vi "Set Bucket RequestPayment Configuration.vi"(4 "Region":T1, 7 "RequestPayment Configuration":T2, 8 "error in (no error)":errorcluster, 9 "Bucket":string) -> (0 "error out":errorcluster)   [LabVIEW 2015, in "LV Interface for Amazon S3.lvlib"]
doc: "This operation <B>sets the RequestPayment configuration</B> of a bucket. By default, <B>the bucket owner pays for downloads from the bucket</B>. This configuration parameter enables the bucket owner (only) to specify that the person requesting the download will be charged for the download."
uses:
  LV Interface for Amazon S3.lvlib
  Typedefs/AMZ_S3_API_RequestPaymentConfig.ctl
  Typedefs/AMZ_S3_Payer.ctl
  Typedefs/AMZ_S3_LocationConstraint.ctl
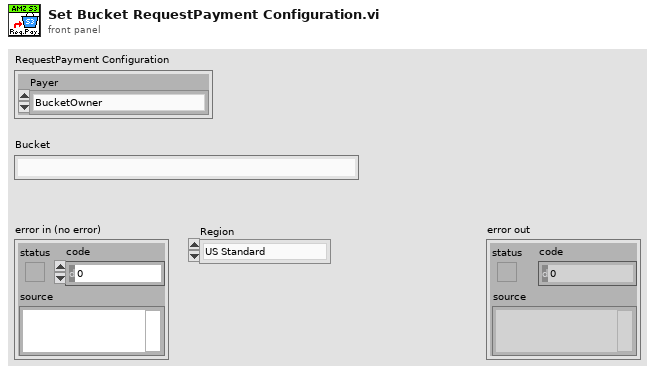
[diagram p1: front panel]
types:
  T1 = typedef "LV Interface for Amazon S3.lvlib/AMZ_S3_LocationConstraint.ctl" = enum16{"US Standard", "us-east-2", "us-west-1", "us-west-2", "ap-northeast-1", "ap-northeast-2", "ap-southeast-1", "ap-southeast-2", "ca-central-1", "eu-central-1", "eu-west-1", "eu-west-2", "sa-east-1"}
  T2 = typedef "LV Interface for Amazon S3.lvlib/AMZ_S3_API_RequestPaymentConfig.ctl" = cluster{"Payer":T3}
  T3 = typedef "LV Interface for Amazon S3.lvlib/AMZ_S3_Payer.ctl" = enum16{"BucketOwner", "Requester"}
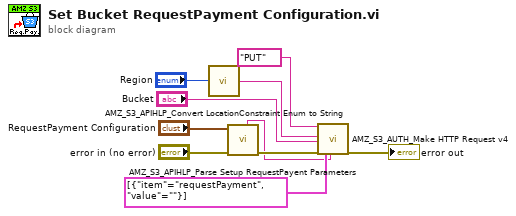
[diagram p0: block diagram]
diagram:
  n1 = call "AMZ_S3_APIHLP_Convert LocationConstraint Enum to String.vi"("Location"="Region") -> ("Location String"=w1:string)  [unwired: 4 in]
  n2 = call "AMZ_S3_APIHLP_Parse Setup RequestPayent Parameters.vi"("error in (no error)"="error in (no error)", "RequestPaymentConfiguration"="RequestPayment Configuration") -> ("error out"=w6:errorcluster, "PUT Data"=w5:string)  [unwired: 8 in]
  n3 = call "AMZ_S3_AUTH_Make HTTP Request v4.vi"("HTTP-Verb"="PUT", "Region"=w1, "Bucket"="Bucket", "error in"=w6, "request parameters"=cluster{"item":string, "value":string}[] [{"item"="requestPayment", "value"=""}], "request body"=w5) -> ("error out"=→"error out":errorcluster)  [unwired: 10 in, 3 out]
